vi "HGCROC Glue Testing.vi"   [LabVIEW 2016]
uses:
  Classes/Workspace/Carrier Tray/Assembly Tray.lvclass
  Classes/Routine/Dispense/CAD Dispense/8 Inch CAD Dispense.lvclass
  Classes/Controller/Controller.lvclass
types:
  T1 = typedef "Controller.lvclass/Controllers.ctl" = cluster{"I-O.lvclass":refnum<class "I-O.lvclass">, "Motion.lvclass":refnum<class "Motion.lvclass">, "Dispenser.lvclass":refnum<class "Dispenser.lvclass">}
  T2 = typedef "Fixture.lvclass/Workspace.ctl" = cluster{"XYZTheta":dbl[], "Workspace Valve":i32, "Workspace Sensor":i32}
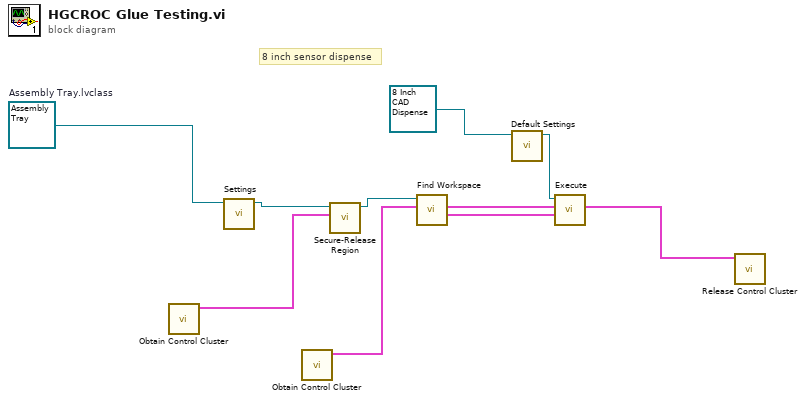
[diagram p0: block diagram]
diagram:
  w10 = refnum<class "Assembly Tray.lvclass"> refnum  # Assembly Tray.lvclass
  # "8 inch sensor dispense"
  n1 = call "Obtain Control Cluster.vi"() -> ("Control Out"=w1:T1)  [unwired: 11 in]
  n2 = call-dynamic "Settings.vi"("Assembly Tray In"=w10) -> ("Assembly Tray Out"=w3:refnum<class "Assembly Tray.lvclass">)  [unwired: 9 in, 1 out]
  n3 = call "Obtain Control Cluster.vi"() -> ("Control Out"=w9:T1)  [unwired: 11 in]
  n4 = call-dynamic "Secure-Release Region.vi"("Control In"=w1, "Carrier Tray in"=w3) -> ("Carrier Tray out"=w2:refnum<class "Assembly Tray.lvclass">)  [unwired: 7 in, 2 out]
  n5 = call-dynamic "Find Workspace.vi"("Control In"=w9, "Carrier Tray in"=w2) -> ("Workspace"=w6:T2, "Control Out"=w5:T1)  [unwired: 6 in, 2 out]
  n6 = call-dynamic "Default Settings.vi"("8 Inch CAD Dispense in"=refnum<class "8 Inch CAD Dispense.lvclass"> refnum ("8 Inch CAD Dispense.lvclass")) -> ("8 Inch CAD Dispense out"=w7:refnum<class "8 Inch CAD Dispense.lvclass">)  [unwired: 9 in, 1 out]
  n7 = call-dynamic "Execute.vi"("Workspace"=w6, "Control In"=w5, "Dispense in"=w7) -> ("Control Out"=w4:T1)  [unwired: 6 in, 2 out]
  n8 = call "Release Control Cluster.vi"("output cluster"=w4) -> ()  [unwired: 11 in]
